vi "SR_Map_Draw.vi"(10 "XY Graph":refnum<vi>, 11 "RDS State in":refnum<class "RDS State.lvclass">) -> ()   [LabVIEW 2015]
uses:
  RDS State Tracker/RDS State/RDS State.lvclass
  Libraries/3rd Party/NMEA_GPS/NMEA_GPRMC-data.ctl
  Libraries/3rd Party/NMEA_GPS/NMEA_LatitudeDirection.ctl
  Libraries/3rd Party/NMEA_GPS/NMEA_LongitudeDirection.ctl
  RDS State Tracker/RDS State/RDS State.lvclass/RDS State.ctl
  Libraries/3rd Party/NMEA_GPS/NMEA.lvlib
panel:
  out "GPRMC-data":T1={"TimeStamp"=timestamp(0 s since 1904-01-01), "Validity"=FALSE, "Latitude"=0.0, "Latitude-Direction"=enum."North", "Longitude"=0.0, "Longitude-Direction"=enum."East", "Speed in knots"=0.0, "True course"=0.0, "Date Stamp"=timestamp(0 s since 1904-01-01), "Magnetic Variation (East/West)"=0.0, "GPS Latitude"=0.0, "GPS Longitude"=0.0} {"GPS Longitude" format="%.6f"; "GPS Latitude" format="%.6f"; "Magnetic Variation (East/West)" format="%.02f [deg]"; "Date Stamp" format="%<%x>T"; "True course" format="%.02f [deg]"; "Speed in knots" format="%.02f [kts]"; "Longitude" format="%0.4f [long]"; "Latitude" format="%.04f [lat]"; "TimeStamp" format="%<%.2X>T"}
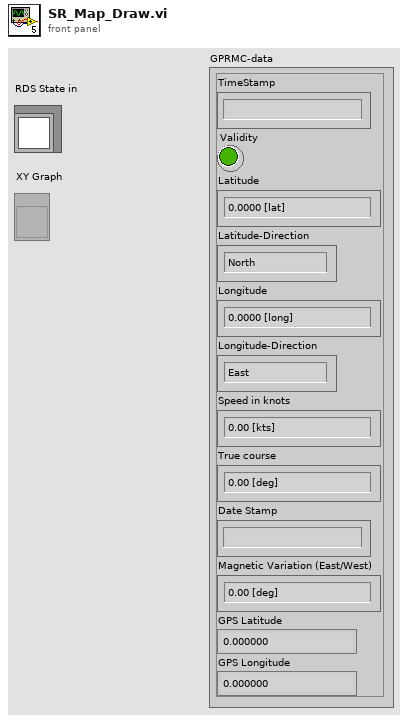
[diagram p1: front panel]
types:
  T1 = typedef "RDS Libraries.lvlib/NMEA.lvlib/NMEA_GPRMC-data.ctl" = cluster{"TimeStamp":timestamp, "Validity":bool, "Latitude":dbl, "Latitude-Direction":T2, "Longitude":dbl, "Longitude-Direction":T3, "Speed in knots":sgl, "True course":sgl, "Date Stamp":timestamp, "Magnetic Variation (East/West)":sgl, "GPS Latitude":dbl, "GPS Longitude":dbl}
  T2 = typedef "RDS Libraries.lvlib/NMEA.lvlib/NMEA_LatitudeDirection.ctl" = enum16{"", "North", "South"}
  T3 = typedef "RDS Libraries.lvlib/NMEA.lvlib/NMEA_LongitudeDirection.ctl" = enum16{"", "East", "West"}
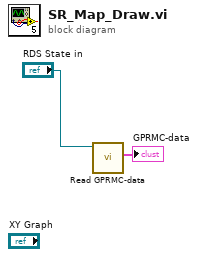
[diagram p0: block diagram]
diagram:
  n1 = call "Read GPRMC-data.vi"("RDS State in"="RDS State in") -> ("GPRMC-data"=→"GPRMC-data":T1)  [unwired: 8 in, 2 out]
